vi "InitialDelta6221_ver2.0.vi"(2 "NV2182A range (V)":dbl=0.01, 4 "Keithley6221 Compliance (V)":dbl=10.0, 5 "Unit":string(combo)="V", 6 "Delay In (s)":dbl, 7 "# of pts discarded":i32=3, 8 "error in (no error)":errorcluster, 9 "Low Level In (A)":dbl, 10 "High Level In (A)":dbl, 11 "VISA Refnum in":refnum<visa-resource-name>) -> (0 "error out":errorcluster, 3 "VISA Refnum out":refnum<visa-resource-name>)   [LabVIEW 2012]
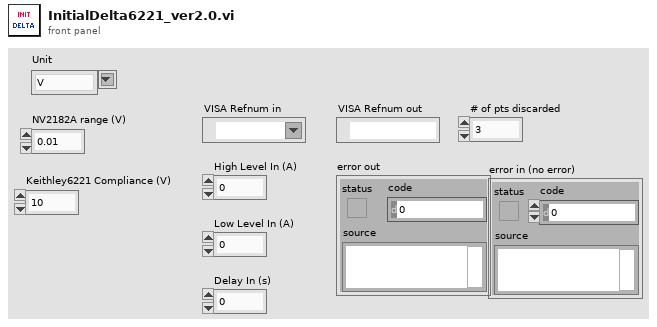
[diagram p1: front panel]
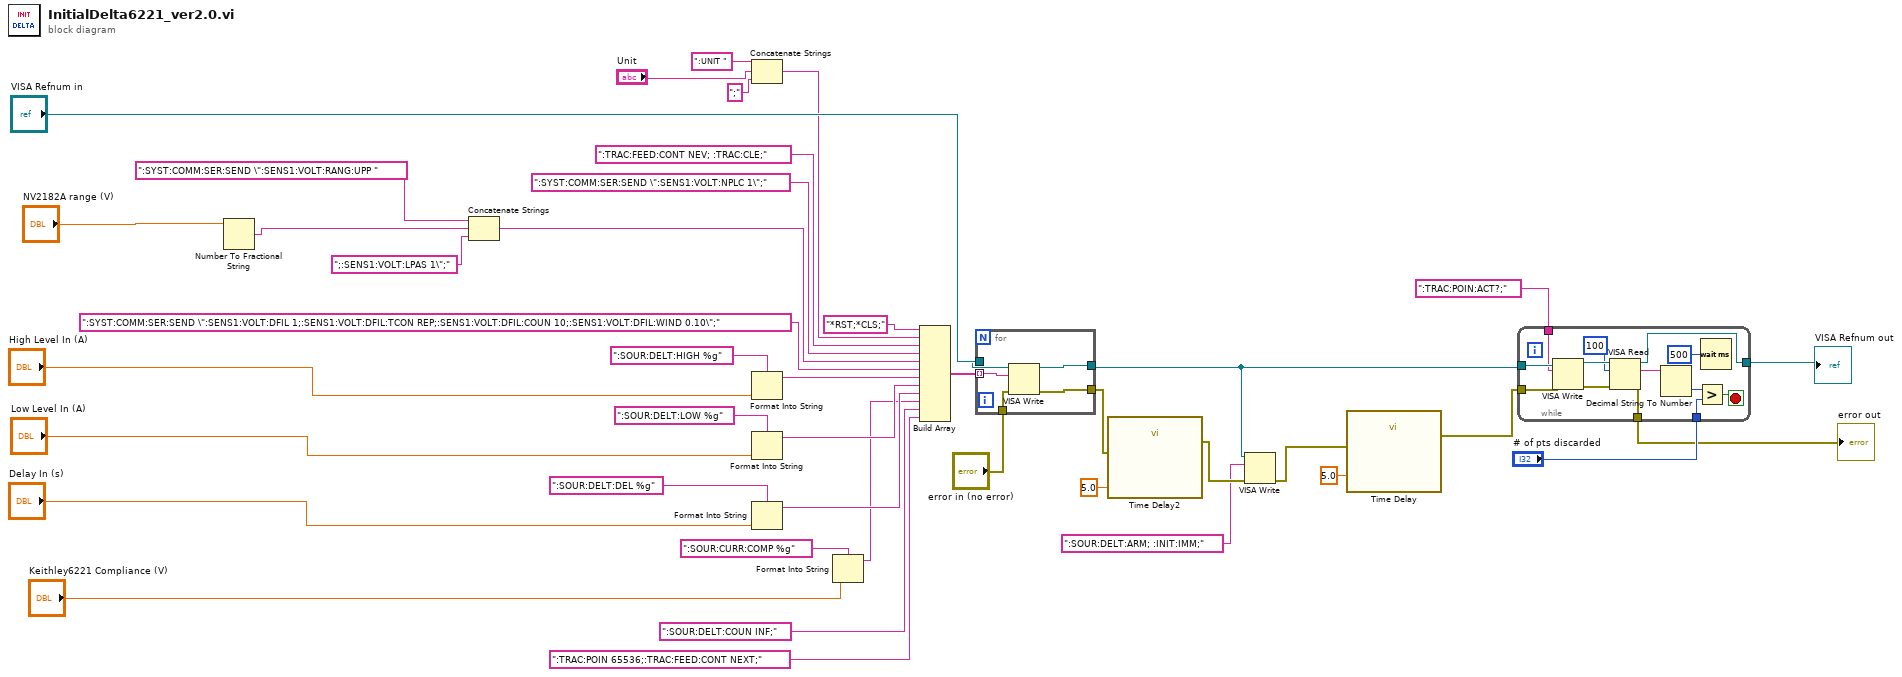
[diagram p0: block diagram]
diagram:
  n1 = Number To Fractional String(number="NV2182A range (V)") -> (F-format string=w6:string)  [unwired: 3 in]
  n2 = Concatenate Strings(":SYST:COMM:SER:SEND \":SENS1:VOLT:RANG:UPP " ("format string"), w6, ";:SENS1:VOLT:LPAS 1\";" ("format string")) -> (w4:string)
  n3 = Concatenate Strings(":UNIT " ("write buffer"), "Unit", ";" ("string")) -> (w9:string)
  n4 = Format Into String(format string=":SOUR:DELT:HIGH %g", "High Level In (A)") -> (resulting string=w33:string)  [unwired: 2 in, 1 out]
  n5 = Format Into String(format string=":SOUR:DELT:LOW %g", "Low Level In (A)") -> (resulting string=w34:string)  [unwired: 2 in, 1 out]
  n6 = Format Into String(format string=":SOUR:DELT:DEL %g", "Delay In (s)") -> (resulting string=w35:string)  [unwired: 2 in, 1 out]
  n7 = Format Into String(format string=":SOUR:CURR:COMP %g", "Keithley6221 Compliance (V)") -> (resulting string=w1:string)  [unwired: 2 in, 1 out]
  n8 = Build Array("*RST;*CLS;" ("write buffer"), w9, ":TRAC:FEED:CONT NEV; :TRAC:CLE;" ("format string"), ":SYST:COMM:SER:SEND \":SENS1:VOLT:NPLC 1\";", w4, ":SYST:COMM:SER:SEND \":SENS1:VOLT:DFIL 1;:SENS1:VOLT:DFIL:TCON REP;:SENS1:VOLT:DFIL:COUN 10;:SENS1:VOLT:DFIL:WIND 0.10\";", w33, w34, w35, w1, ":SOUR:DELT:COUN INF;", ":TRAC:POIN 65536;:TRAC:FEED:CONT NEXT;" ("format string")) -> (w38:string[])
  n9 = for {
    tunnel: w38 -> [w47] mode=indexing
    tunnel: "VISA Refnum in" -> [w46]
    tunnel: [w45] -> w16
    tunnel: [w44] -> w18
    tunnel: "error in (no error)" -> [w43]
    n10 = VISA Write(VISA resource name=w46, write buffer=w47, error in (no error)=w43) -> (VISA resource name out=w45:refnum<visa-resource-name>, error out=w44:errorcluster)  [unwired: 1 out]
  }
  n11 = call "Time Delay2"("error in (no error)"=w18, "Delay Time (s)"=5.0) -> ("error out"=w17:errorcluster)  [unwired: 9 in]
  n12 = VISA Write(VISA resource name=w16, write buffer=":SOUR:DELT:ARM; :INIT:IMM;" ("format string"), error in (no error)=w17) -> (error out=w14:errorcluster)  [unwired: 2 out]
  n13 = call "Time Delay"("error in (no error)"=w14, "Delay Time (s)"=5.0) -> ("error out"=w20:errorcluster)  [unwired: 9 in]
  n14 = while {
    tunnel: w16 -> [w60]
    tunnel: w20 -> [w59]
    tunnel: ":TRAC:POIN:ACT?;" ("write buffer") -> [w58]
    tunnel: [w51] -> w22
    tunnel: "# of pts discarded" -> [w49]
    tunnel: [w48] -> w21
    stop <- w52 stop-if-true
    n15 = VISA Write(VISA resource name=w60, write buffer=w58, error in (no error)=w59) -> (VISA resource name out=w56:refnum<visa-resource-name>, error out=w57:errorcluster)  [unwired: 1 out]
    n16 = VISA Read(VISA resource name=w56, byte count=u32 100, error in (no error)=w57) -> (VISA resource name out=w48:refnum<visa-resource-name>, read buffer=w54:string, error out=w51:errorcluster)  [unwired: 1 out]
    n17 = Decimal String To Number(string=w54) -> (number=w53:i32)  [unwired: 2 in, 1 out]
    n18 = Greater?(x=w53, y=w49) -> (0:w52:bool)
    n19 = Wait (ms)(milliseconds to wait=u32 500) -> ()  [unwired: 1 out]
  }
  "error out" <- w22
  "VISA Refnum out" <- w21
